vi "Check Loop Status.vi"(8 "Error in":errorcluster, 11 "State Variables in":T1={"Stop Notifier"=refnum, "UI References"=[], "DAQmx"={"ECG Input"={"Channel"="", "Task"="", "Max Value"=0.0, "Min Value"=0.0, "Sampling Rate"=0.0, "Batch Size"=0}, "Trigger Output"={"Channel"="", "Task"="", "Pulse Frequency"=0.0, "Delay"=0, "Triggers per Shot"=0}}, "Data Queue"=refnum, "Filter"={"Batch Size"=1000, "Update Cycle"=0, "Filter Buffer"=[]}, "Last Detect Result"=FALSE}) -> (0 "Error out":errorcluster, 2 "Stop Loop?":bool, 3 "State Variables out":T1={"Stop Notifier"=refnum, "UI References"=[], "DAQmx"={"ECG Input"={"Channel"="", "Task"="", "Max Value"=0.0, "Min Value"=0.0, "Sampling Rate"=0.0, "Batch Size"=0}, "Trigger Output"={"Channel"="", "Task"="", "Pulse Frequency"=0.0, "Delay"=0, "Triggers per Shot"=0}}, "Data Queue"=refnum, "Filter"={"Batch Size"=1000, "Update Cycle"=0, "Filter Buffer"=[]}, "Last Detect Result"=FALSE})   [LabVIEW 2014, in "Flow Control.lvlib"]
uses:
  Flow Control.lvlib
  Controls/State Variables.ctl
  Controls/DAQmx Variables.ctl
  Controls/Filter Variables.ctl
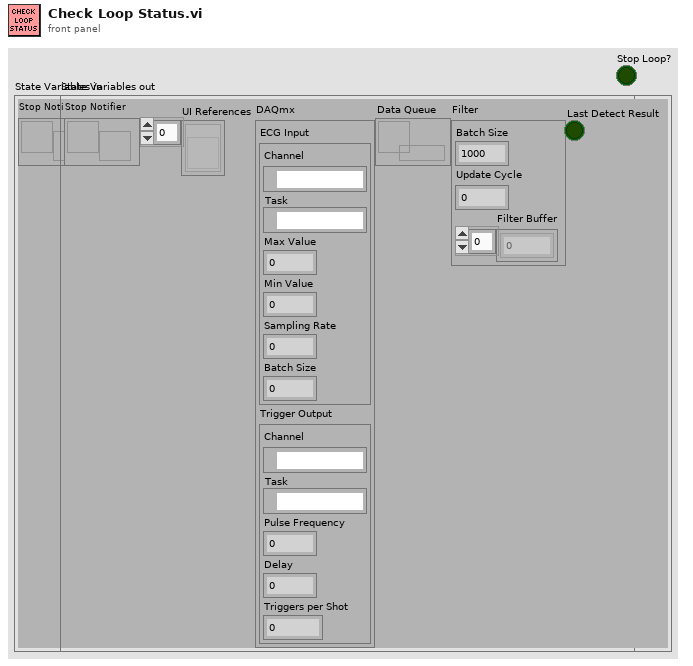
[diagram p1: front panel]
types:
  T1 = typedef "State Variables.ctl" = cluster{"Stop Notifier":refnum<notifier>, "UI References":refnum<vi>[], "DAQmx":T2, "Data Queue":refnum<queue>, "Filter":T3, "Last Detect Result":bool}
  T2 = typedef "DAQmx Variables.ctl" = cluster{"ECG Input":cluster{"Channel":tag, "Task":refnum<k21>, "Max Value":dbl, "Min Value":dbl, "Sampling Rate":dbl, "Batch Size":i32}, "Trigger Output":cluster{"Channel":tag, "Task":refnum<k21>, "Pulse Frequency":dbl, "Delay":u16, "Triggers per Shot":i32}}
  T3 = typedef "Filter Variables.ctl" = cluster{"Batch Size":i32, "Update Cycle":i32, "Filter Buffer":dbl[]}
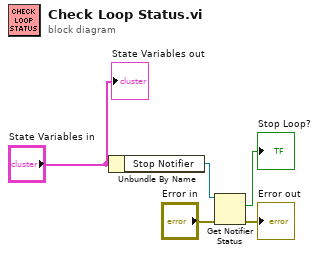
[diagram p0: block diagram]
diagram:
  n1 = Unbundle By Name("State Variables in") -> ("Stop Notifier"=w4:refnum<notifier>)
  n2 = Get Notifier Status(notifier=w4, error in (no error)="Error in") -> (current notification=→"Stop Loop?":bool, error out=→"Error out":errorcluster)  [unwired: 3 out]
  "State Variables out" <- "State Variables in"
